vi "sendCommand.vi"(8 "error in (no error)":errorcluster, 9 "Read?":bool, 10 "command":string, 11 "Telnet in":refnum<class "Telnet.lvclass">) -> (0 "error out":errorcluster, 2 "reply":string, 3 "Telnet out":refnum<class "Telnet.lvclass">)   [LabVIEW 2011, in "Hardware.lvlib" / "HWControllers.lvlib" / "Telnet.lvclass"]
uses:
  Telnet.lvclass
  Telnet.lvclass/Telnet.ctl
  <vilib>/addons/internet/NI_InternetTK_Core_VIs.lvlib
panel:
  out "bytes written":i32
  in  "stop":bool
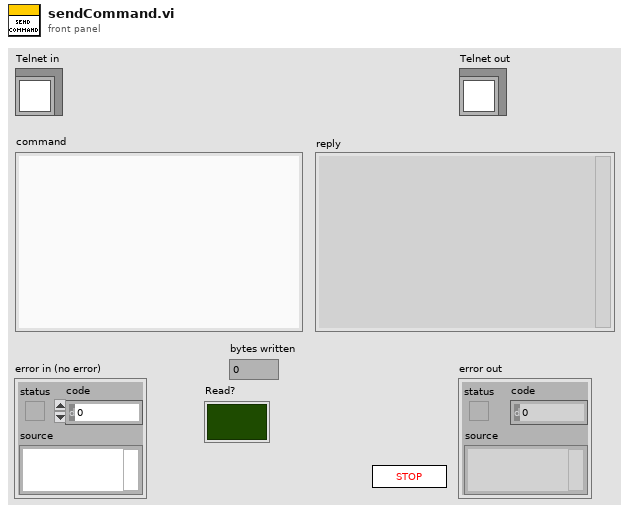
[diagram p1: front panel]
types:
  T1 = typedef "Telnet Session.ctl" = refnum<k1>
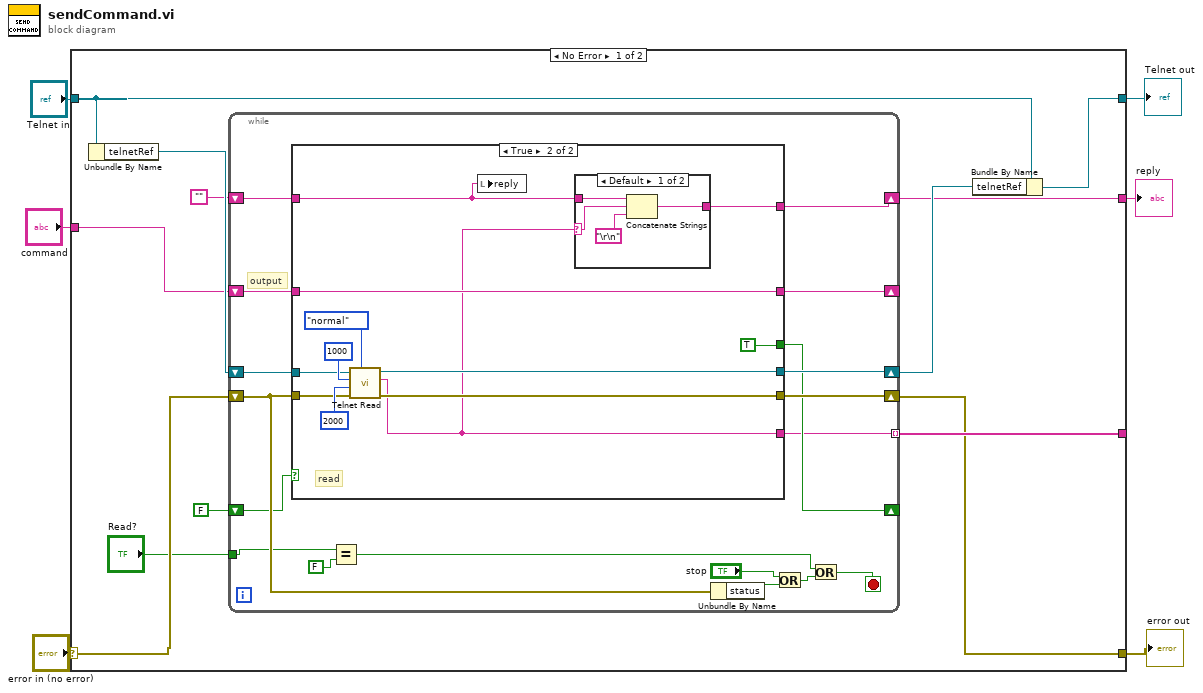
[diagram p0: block diagram]
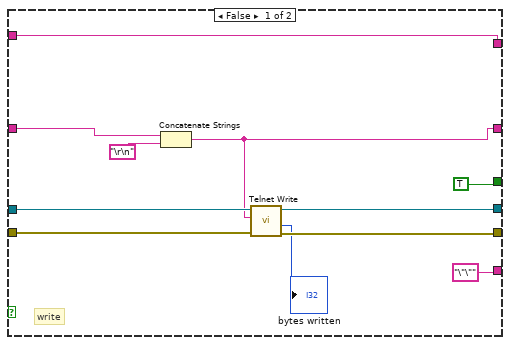
[diagram p2: hidden frame]
diagram:
  n1 = case shown="No Error" "error in (no error)" {
    selector: "error in (no error)" -> [w16 w66]
    tunnel: [w15 w66] -> w5
    tunnel: [w12 w65] -> w3
    tunnel: "Telnet in" -> [w13 w65]
    tunnel: "command" -> [w10 _]
    tunnel: [w17 _] -> _
    tunnel: [w8 _] -> w1
    frame No Error {
      n2 = Unbundle By Name(w13) -> ("telnetRef"=w14:T1)
      n3 = while {
        shift-right: [w35] -> w11
        shift-left: w14 -> [w36]
        shift-right: [w34] -> w15
        shift-left: w16 -> [w31]
        shift-right: [w29] -> _
        shift-left: w10 -> [w30]
        shift-right: [w27] -> _
        shift-left: FALSE -> [w28]
        tunnel: [w26] -> w17 mode=indexing
        shift-right: [w24] -> w8
        shift-left: "" -> [w25]
        tunnel: "Read?" -> [w23]
        stop <- w19 stop-if-true
        # "output"
        n4 = case shown="True" w28 {
          tunnel: w36 -> [w46 w57]
          tunnel: [w43 w56] -> w35
          tunnel: [w44 w55] -> w34
          tunnel: w31 -> [w45 w54]
          tunnel: w30 -> [w41 w53]
          tunnel: [w39 w53] -> w29
          tunnel: [TRUE TRUE] -> w27
          tunnel: ["\"\"" w50] -> w26
          tunnel: w25 -> [w37 w48]
          tunnel: [w37 w49] -> w24
          frame False {
            # "write"
            n5 = Concatenate Strings(w41, "\r\n") -> (w39:string)
            n6 = call <vilib>:"Telnet Write.vi"("error in (no error)"=w45, "data in"=w39, "telnet connection"=w46) -> ("error out"=w44:errorcluster, "bytes written"=→"bytes written":i32, "telnet connection out"=w43:T1)  [unwired: 4 in]
          }
          frame True {
            # "read"
            n7 = call <vilib>:"Telnet Read.vi"("read mode (normal)"=enum16{"normal", "line", "buffered"}."normal", "error in (no error)"=w54, "timeout ms (25000)"=2000, "bytes to read"=1000, "telnet connection"=w57) -> ("error out"=w55:errorcluster, "data out"=w50:string, "telnet connection out"=w56:T1)  [unwired: 2 out]
            n8 = local write "reply"(w48) -> ()
            n9 = case shown="Default" w50 {
              selector: w50 -> [w62 _]
              tunnel: w48 -> [w63 w64]
              tunnel: [w60 w64] -> w49
              frame Default {
                n10 = Concatenate Strings(w63, w62, "\r\n") -> (w60:string)
              }
              frame "\u0000" {
              }
            }
          }
        }
        n11 = Equal?(x=w23, y=FALSE) -> (x = y?=w20:bool)
        n12 = Unbundle By Name(w31) -> ("status"=w32:bool)
        n13 = Or(x="stop", y=w32) -> (x .or. y?=w21:bool)
        n14 = Or(x=w20, y=w21) -> (x .or. y?=w19:bool)
      }
      n15 = Bundle By Name(cluster=w13, "telnetRef"=w11) -> (w12:refnum<class "Telnet.lvclass">)
    }
    frame Error {
    }
  }
  "error out" <- w5
  "Telnet out" <- w3
  "reply" <- w1
